vi "Colour_Hardcode.vi"() -> ()   [LabVIEW 2017]
panel:
  out "green":bool
  out "total sum":u8
  out "yellow":bool
  out "black":bool
  in  "A/12C":tag="B/I2C"
  in  "Start":bool
  out "Loops":i32
  in  "Stop":bool
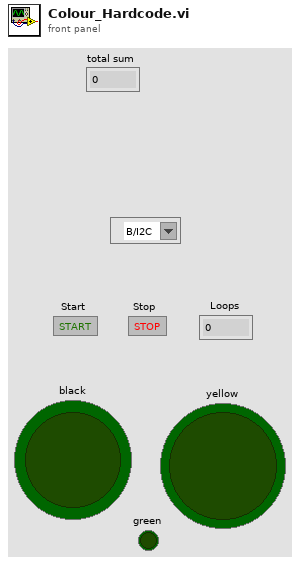
[diagram p1: front panel]
types:
  T1 = typedef "I2C.lvlib/I2C Reference.ctl" = cluster{"myRIO Reference":T2, "I2C Channels Enum":T6, "I2C Configuration":T7}
  T2 = typedef "myRIO Generic Hardware Reference.ctl" = cluster{"myRIO Model":T3, "myRIO Hardware Reference":T4}
  T3 = typedef "Hardware Version Enum.ctl" = enum16{"Unknown", "myRIO-1900", "myRIO-1950", "roboRIO", "NI ELVIS RIO CM"}
  T4 = typedef "myRIO v1.0 Reference.ctl" = cluster{"Generic FPGA Reference":T5, "Allow multiple opens":bool}
  T5 = typedef "Generic FPGA Reference.ctl" = refnum<k20>
  T6 = typedef "I2C Channels Enum.ctl" = enum16{"Not Connected", "A/I2C", "B/I2C", "I2C/I2C"}
  T7 = typedef "I2C.lvlib/I2C Configuration.ctl" = cluster{"I2C Transfer Rate":T8}
  T8 = typedef "I2C.lvlib/I2C Transfer Rate.ctl" = enum16{"Standard mode (100 kbps)", "Fast mode (400 kbps)"}
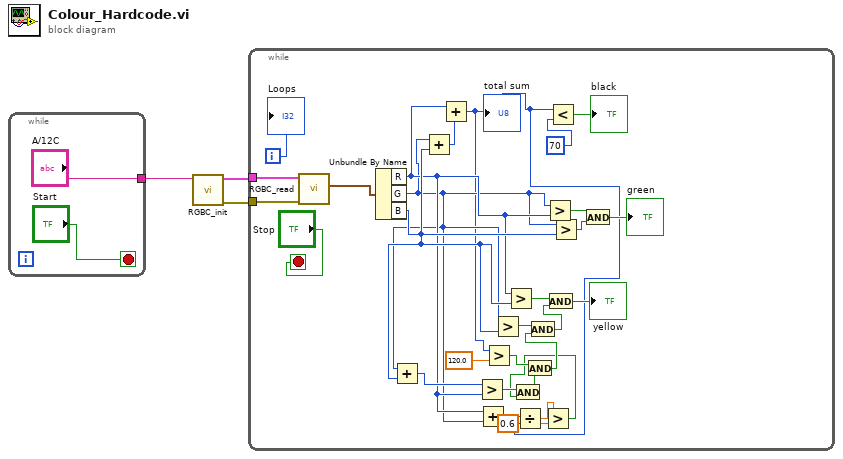
[diagram p0: block diagram]
diagram:
  n1 = while {
    tunnel: ["A/12C"] -> w2
    stop <- "Start" stop-if-true
  }
  n2 = call "RGBC_init.vi"("Channel Name"=w2) -> ("error out"=w3:errorcluster, "I2C Ref Out"=w1:T1)  [unwired: 9 in]
  n3 = while {
    tunnel: w3 -> [w34]
    tunnel: w1 -> [w33]
    i -> [w31]
    stop <- "Stop" stop-if-true
    n4 = call "RGBC_read.vi"("error in (no error)"=w34, "I2C Ref In"=w33) -> ("RGB"=w30:cluster{"R":u8, "G":u8, "B":u8})  [unwired: 7 in, 2 out]
    n5 = Unbundle By Name(w30) -> ("R"=w12:u8, "G"=w11:u8, "B"=w16:u8)
    n6 = Add(x=w11, y=w16) -> (x+y=w19:u8)
    n7 = Add(x=w11, y=w16) -> (x+y=w29:u8)
    n8 = Add(x=w12, y=w29) -> (x+y=w9:u8)
    "total sum" <- w9
    n9 = Greater?(x=w19, y=w12) -> (0:w13:bool)
    n10 = Add(x=w12, y=w11) -> (x+y=w10:u8)
    n11 = Greater?(x=w9, y=120.0) -> (0:w21:bool)
    n12 = Greater?(x=w11, y=w16) -> (0:w23:bool)
    n13 = Greater?(x=w12, y=w16) -> (0:w27:bool)
    n14 = Divide(x=w10, y=w9) -> (x/y=w8:dbl)
    n15 = Greater?(x=w8, y=0.6) -> (0:w6:bool)
    n16 = And(x=w13, y=w6) -> (x .and. y?=w14:bool)
    n17 = And(x=w21, y=w14) -> (x .and. y?=w20:bool)
    n18 = And(x=w23, y=w20) -> (x .and. y?=w24:bool)
    n19 = Greater?(x=w11, y=w12) -> (0:w18:bool)
    n20 = And(x=w27, y=w24) -> (x .and. y?=→"yellow":bool)
    n21 = Less?(x=w9, y=u8 70) -> (x < y?=→"black":bool)
    n22 = Greater?(x=w11, y=w16) -> (0:w17:bool)
    n23 = And(x=w18, y=w17) -> (x .and. y?=→"green":bool)
    "Loops" <- w31
  }
